vi "CC Script Parsing Test.vi"() -> ()   [LabVIEW 2020]
panel:
  out "Script Ok?":bool
  out "Script String":string
  in  "Script text":string="DefineObject Alpha1234 \"Type\":\"Standard\",\"RA\":\"123.456\",\"DEC\":456.789\"\nDefineExposure Exp1 \"Number\":\"1\",\"Groups\":\"1\",\"ReadoutsPerGroup\":\"1\",\"TimeBetweenGroups\":\"10\",\"TimeBetweenReadouts\":\"10\"\nDefineDithering Dither2 \"Offsets\":\"(0,0),(-10,-10)\"\nFilterWheel (A,B)\nAcquireImages (Alpha1234,Exp1,Dither2)\n"
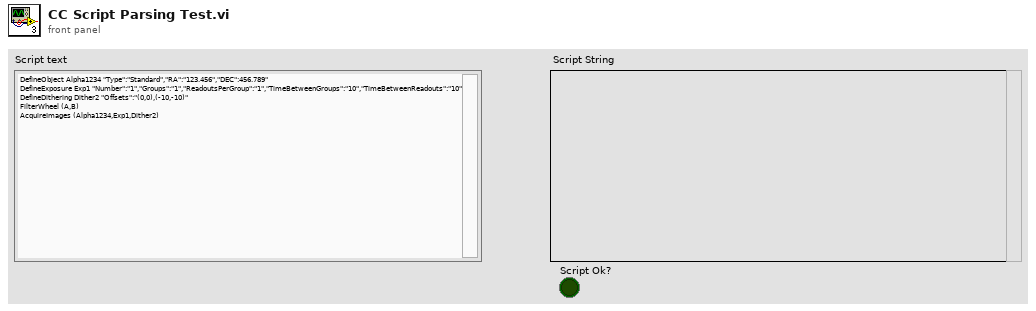
[diagram p1: front panel]
types:
  T1 = typedef "CC Script Step.ctl" = cluster{"Action":T2, "Data":variant}
  T2 = typedef "CC enum Script Action.ctl" = enum16{"Noop", "Define Object", "Define Exposure", "Define Dithering", "Acquire Images", "Set Filter Wheel", "Telescope Home", "Telescope Move", "Focus Move Relative", "Focus Move Absolute", "Focus Set Home", "Macro", "Pause", "Ask User", "Define Random Dither"}
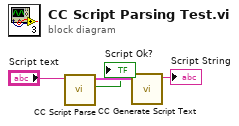
[diagram p0: block diagram]
diagram:
  n1 = call "CC Script Parse.vi"("Script text"="Script text") -> ("Script Ok?"=→"Script Ok?":bool, "Script steps"=w3:T1[])  [unwired: 7 in, 2 out]
  n2 = call "CC Generate Script Text.vi"("Script"=w3) -> ("Script String"=→"Script String":string)  [unwired: 9 in, 1 out]
